vi "File_CreateFolders.vi"(1 "Path":path, 3 "Promt if folder\ndoes not exists?":bool, 5 "error in (no error)":errorcluster, 6 "permissions (0755)":i16=493 format="%.0o") -> (15 "File permission error!":bool, 16 "Folder exists?":bool, 19 "error out":errorcluster)   [LabVIEW 2020]
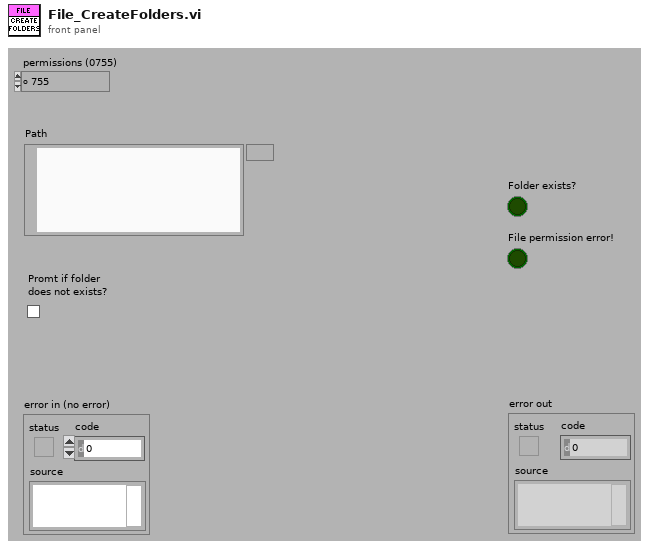
[diagram p1: front panel]
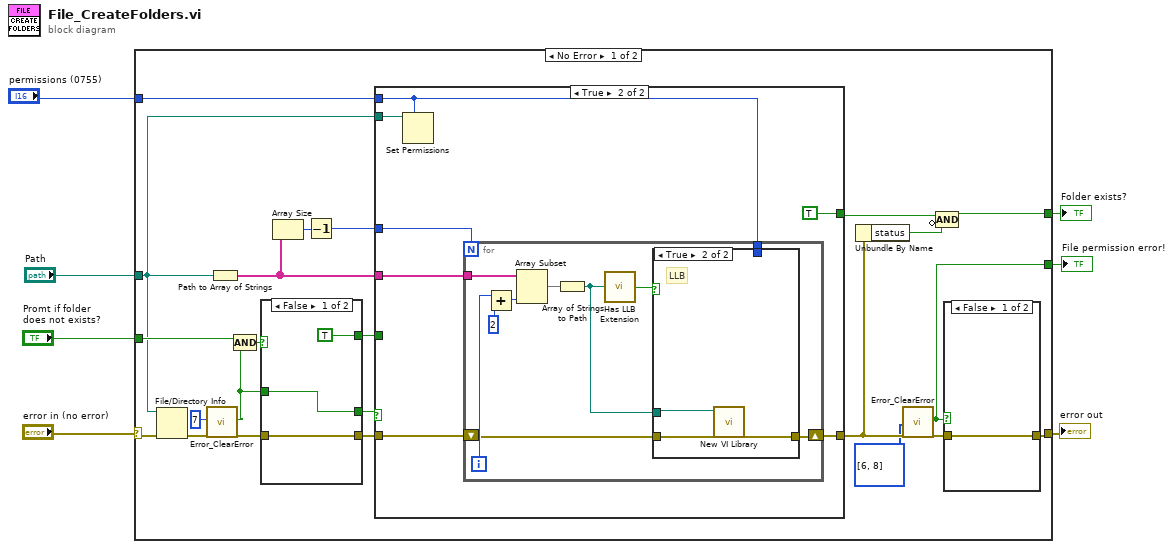
[diagram p0: block diagram]
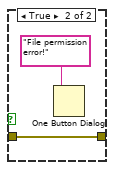
[diagram p2: hidden frame]
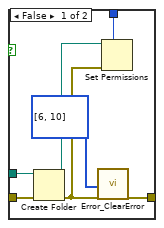
[diagram p4: hidden frame]
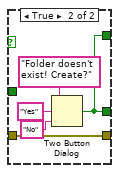
[diagram p5: hidden frame]
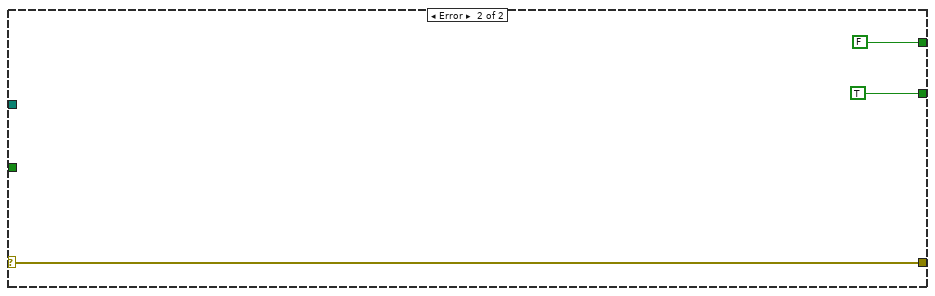
[diagram p6: hidden frame]
diagram:
  n1 = case shown="No Error" "error in (no error)" {
    selector: "error in (no error)" -> [w30 w73]
    tunnel: "Path" -> [w9 _]
    tunnel: [w23 w73] -> w5
    tunnel: [w22 TRUE ("Cleared?")] -> w4
    tunnel: [w18 FALSE] -> w3
    tunnel: "Promt if folder\ndoes not exists?" -> [w15 _]
    tunnel: "permissions (0755)" -> [w8 _]
    frame No Error {
      n2 = File/Directory Info(path=w9, error in=w30) -> (error out=w29:errorcluster)  [unwired: 6 out]
      n3 = call <resource>:"Error_ClearError.vi"("code"=7, "error in (no error)"=w29) -> ("Cleared?"=w14:bool, "error out"=w27:errorcluster)  [unwired: 3 in, 13 out]
      n4 = Path to Array of Strings(0:w9) -> (2:w13:string[])  [unwired: 1 out]
      n5 = Compound Arithmetic op=AND(w15, w14) -> (w16:bool)
      n6 = case shown="False" w16 {
        tunnel: w27 -> [w65 w67]
        tunnel: [w65 w67] -> w25
        tunnel: [w63 w66] -> w26
        tunnel: [TRUE w66] -> w17
        tunnel: w14 -> [w63 _]
        frame False {
        }
        frame True {
          n7 = Two Button Dialog(message="Folder doesn't exist! Create?", 1:"No" ("F button name (\"Cancel\")"), 2:"Yes" ("T button name (\"OK\")")) -> (T button?=w66:bool)
        }
      }
      n8 = Array Size(array=w13) -> (size(s)=w12:i32)
      n9 = Decrement(x=w12) -> (x-1=w11:i32)
      n10 = case shown="True" w26 {
        tunnel: w13 -> [_ w39]
        tunnel: [w35 w42] -> w21
        tunnel: w25 -> [w35 w40]
        tunnel: [w34 TRUE] -> w20
        tunnel: w17 -> [w34 _]
        tunnel: w11 -> [_ w38]
        tunnel: w9 -> [_ w37]
        tunnel: w8 -> [_ w36]
        frame False {
        }
        frame True {
          n11 = Set Permissions(7:w36, 11:w37) -> ()  [unwired: 1 in, 4 out]
          n12 = for {
            N: w38 -> [_]
            shift-right: [w44] -> w42
            shift-left: w40 -> [w46]
            tunnel: w39 -> [w52]
            tunnel: w36 -> [w43]
            i -> [w51]
            n13 = Add(x=w51, y=2) -> (x+y=w50:i32)
            n14 = Array Subset(array=w52, length=w50) -> (w48:string[])  [unwired: 1 in]
            n15 = Array of Strings to Path(0:w48) -> (2:w45:path)  [unwired: 1 out]
            n16 = call <vilib>:"Has LLB Extension.vi"("path"=w45) -> ("path to VI library?"=w47:bool)
            n17 = case shown="True" w47 {
              tunnel: w46 -> [w59 w61]
              tunnel: w45 -> [w58 w60]
              tunnel: [w57 w62] -> w44
              tunnel: w43 -> [w54 _]
              frame False {
                n18 = Create Folder(path (use dialog)=w58, error in=w59) -> (created path=w53:path, error out=w55:errorcluster)  [unwired: 2 out]
                n19 = call <resource>:"Error_ClearError.vi"("codes"=i32[] [6, 10], "error in (no error)"=w55) -> ("error out"=w57:errorcluster)  [unwired: 3 in, 14 out]
                n20 = Set Permissions(7:w54, 8:w55, 11:w53) -> ()  [unwired: 4 out]
              }
              frame True {
                # "LLB"
                n21 = call <vilib>:"New VI Library.vi"("error in (no error)"=w61, "VI library path in"=w60) -> ("error out"=w62:errorcluster)  [unwired: 9 out]
              }
            }
          }
        }
      }
      n22 = Unbundle By Name(w21) -> ("status"=w19:bool)
      n23 = call <resource>:"Error_ClearError.vi"("codes"=i32[] [6, 8], "error in (no error)"=w21) -> ("Cleared?"=w22:bool, "error out"=w24:errorcluster)  [unwired: 3 in, 13 out]
      n24 = Compound Arithmetic op=AND(w20, invert w19) -> (w18:bool)
      n25 = case shown="False" w22 {
        tunnel: w24 -> [w31 w33]
        tunnel: [w31 w33] -> w23
        frame False {
        }
        frame True {
          n26 = One Button Dialog(message="File permission error!") -> ()  [unwired: 2 out]
        }
      }
    }
    frame Error {
    }
  }
  "error out" <- w5
  "File permission error!" <- w4
  "Folder exists?" <- w3
